vi "XYGraphView.vi"() -> ()   [LabVIEW 2014]
uses:
  GlobalData/GlobalXyData.vi
panel:
  in  "btnInitial":bool
  in  "太線(+3)":bool
  in  "自動スケール":bool
  in  "軸本数":u16(ring)=4 items=["２"=2, "４"=4, "６"=6, "８"=8]
  in  "MIN":dbl format="%#_6f"
  in  "MAX":dbl format="%#_6f"
  in  "Y軸":u16(ring) items=["No.", "M1回転rpm", "M2回転rpm", "M3回転rpm", "M1トルクN･m", "M2トルクN･m", "M3トルクN･m", "a"]
  in  "プロットCH":u16(ring) items=["No.", "M1回転rpm", "M2回転rpm", "M3回転rpm", "M1トルクN･m", "M2トルクN･m", "M3トルクN･m", "", "", "", "", "", "", "", "", "", "", "供試体温度1℃", "供試体温度2℃", "供試体温度3℃", "動力盤温度℃", "軸受温度1℃", "軸受温度2℃", "軸受温度3℃", "", "効率"]
  in  "名称":string
  in  "色":u32(colorbox)
  in  "btnAddCursor":bool
  in  "btnScaleLegendVis":bool
  in  "btnLegVis":bool
  in  "btnCursorLegendVis":bool
  out "XYグラフ":cluster{"X配列":dbl[], "Y配列":dbl[]}[](graph)
  # "表示"
  # "カーソル"
  # "グラフCH設定"
  # "右クリック→カーソルを作成→複数プロット。さらに右クリック→監視→全てのプロット"
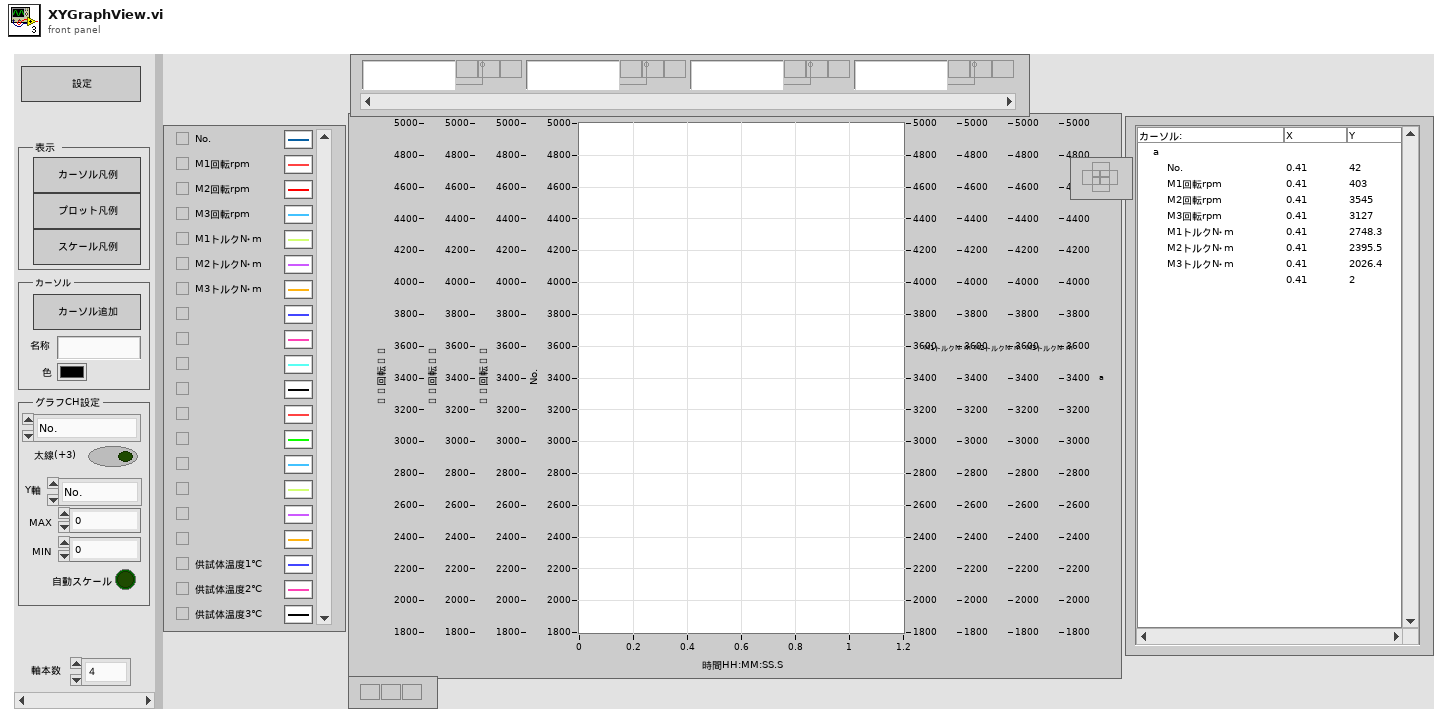
[diagram p1: front panel]
types:
  T1 = typedef "eventvkey.ctl" = enum16{"ASCII", "Enter", "Return", "Shift", "Ctrl", "Alt", "Cmd", "Opt", "Caps", "NumLock", "Clear", "Break", "Up", "Down", "Left", "Right", "Insert", "Delete", "Home", "End", "PageUp", "PageDown", "Escape", "Help", "Pause", "ScrollLock", "F1", "F2", "F3", "F4", "F5", "F6", "F7", "F8", "F9", "F10", "F11", "F12", "F13", "F14", "F15", "F16", "F17", "F18", "F19", "F20", "F21", "F22", "F23", "F24", "Play", "VolumeUp", "VolumeDown", "Mute", "Two Byte Char"}
  T2 = typedef "LVRangeTypeDef.ctl" = cluster{"Minimum":dbl, "Maximum":dbl, "Increment":dbl, "Minor Increment":dbl, "Start":dbl}
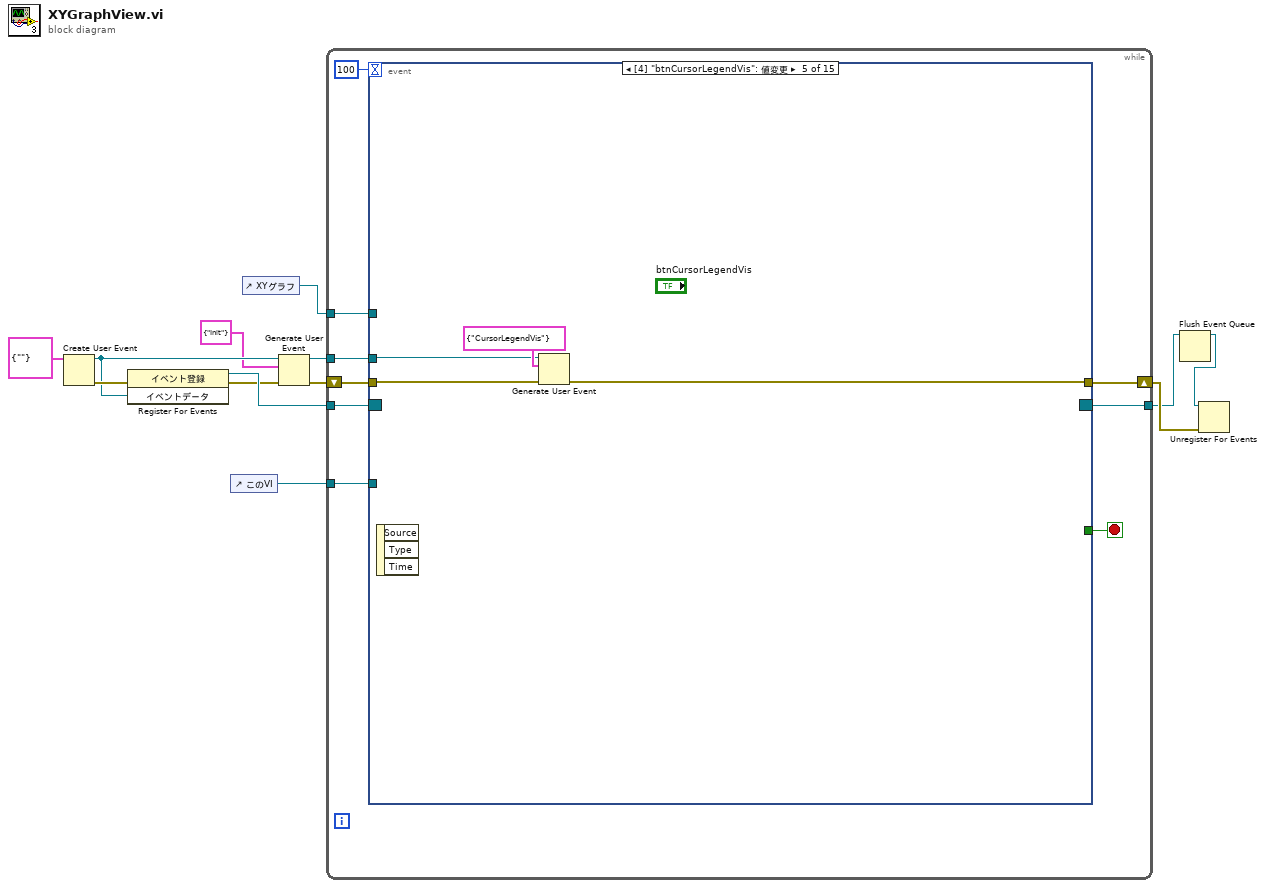
[diagram p0: block diagram]
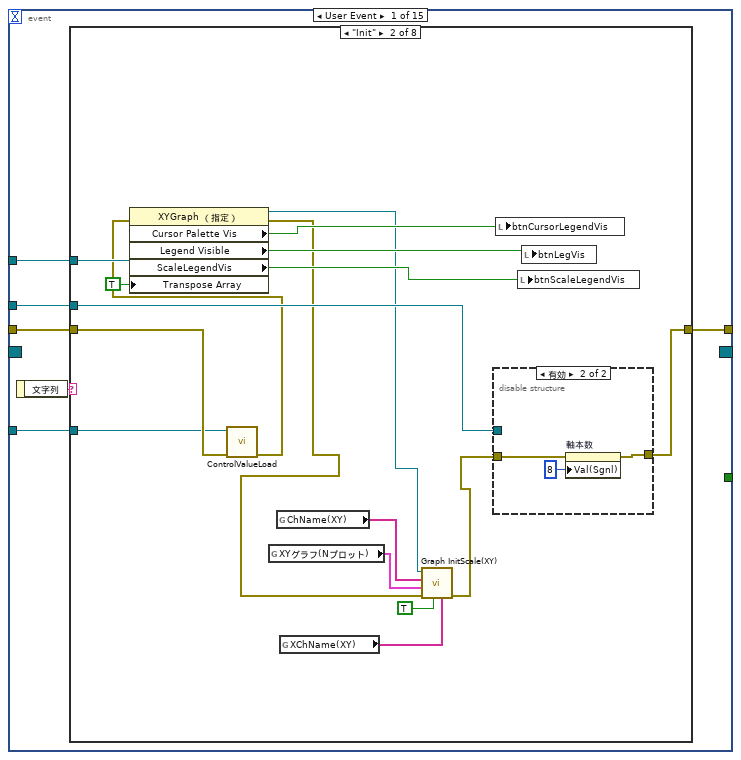
[diagram p2: hidden frame]
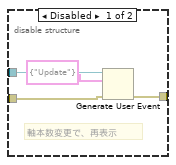
[diagram p4: hidden frame]
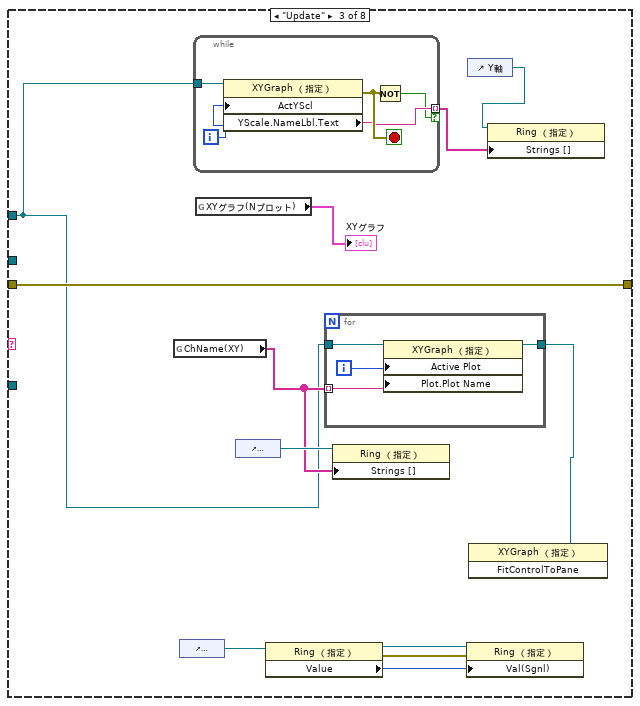
[diagram p5: hidden frame]
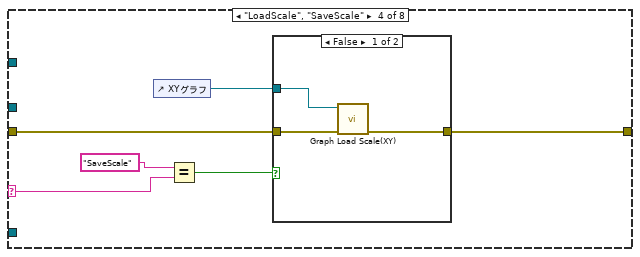
[diagram p6: hidden frame]
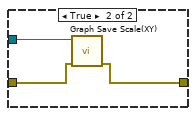
[diagram p7: hidden frame]
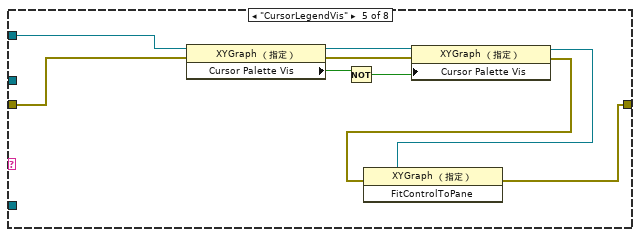
[diagram p8: hidden frame]
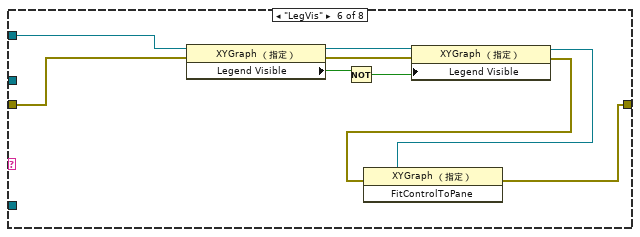
[diagram p9: hidden frame]
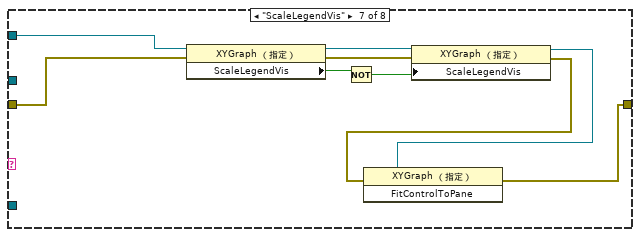
[diagram p10: hidden frame]
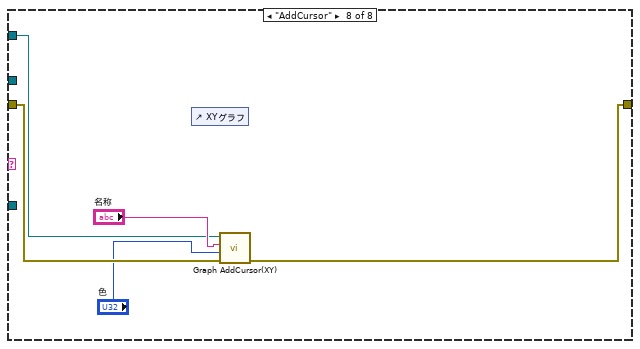
[diagram p11: hidden frame]
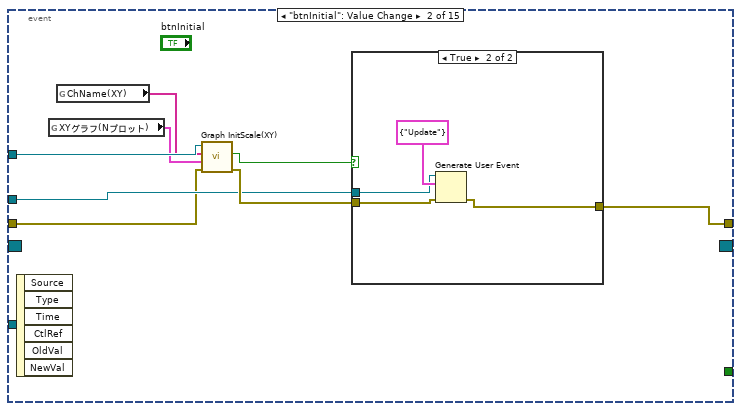
[diagram p12: hidden frame]
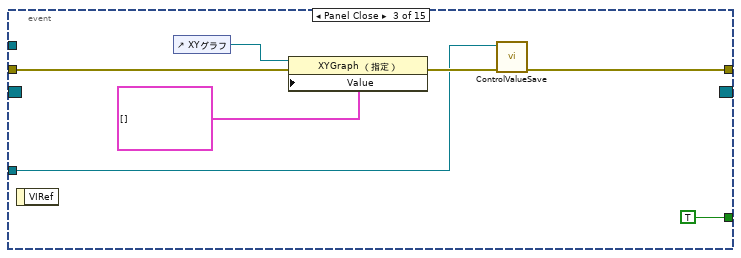
[diagram p14: hidden frame]
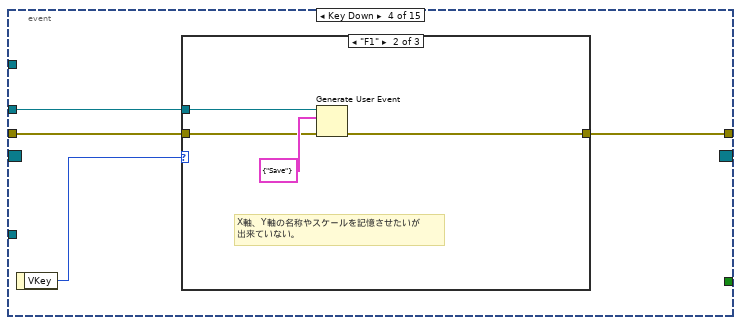
[diagram p15: hidden frame]
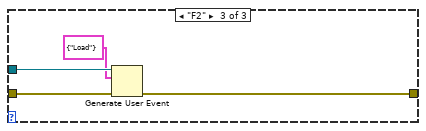
[diagram p17: hidden frame]
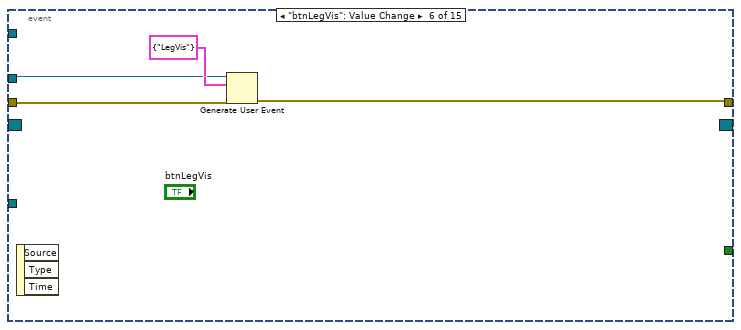
[diagram p18: hidden frame]
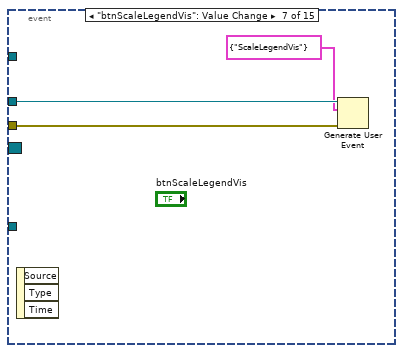
[diagram p19: hidden frame]
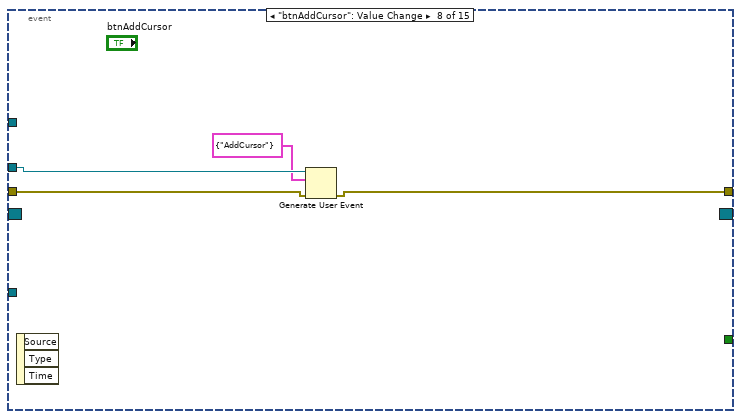
[diagram p20: hidden frame]
diagram:
  n1 = Create User Event(user event datatype=cluster{"文字列":string} {"文字列"=""} ("イベントデータ")) -> (user event=w10:refnum<user-event>, error out=w11:errorcluster)  [unwired: 1 in]
  n2 = register-events(error in=w11, w10) -> (reference out=w13:refnum<event-registration>, error out=w9:errorcluster)  [unwired: 1 in]
  n3 = control-ref of="このVI"() -> (w5:refnum<vi>)
  n4 = control-ref of="XYグラフ"() -> (w3:refnum<vi>)
  n5 = Generate User Event(user event=w10, event data cluster=cluster{"文字列":string} {"文字列"="Init"} ("イベントデータ"), error in=w9) -> (user event out=w6:refnum<user-event>, error out=w8:errorcluster)  [unwired: 1 in]
  n6 = while {
    tunnel: w13 -> [w21]
    tunnel: [w20] -> w2
    tunnel: w6 -> [w19]
    tunnel: w5 -> [w18]
    shift-right: [w16] -> w4
    shift-left: w8 -> [w17]
    tunnel: w3 -> [w15]
    stop <- w22 stop-if-true
    n7 = event shown="[4] \"btnCursorLegendVis\": 値変更" {
      selector: w21 -> [_ _ _ _ _ _ _ _ _ _ _ _ _ _ _]
      dyn-events: [_ _ _ _ _ _ _ _ _ _ _ _ _ _ _] -> w20
      timeout: 100 -> [_ _ _ _ _ _ _ _ _ _ _ _ _ _ _]
      tunnel: [_ _ TRUE _ _ _ _ _ _ _ _ _ _ _ _] -> w22
      tunnel: w19 -> [w27 w124 _ w141 w153 w158 w162 w166 _ _ _ _ w208 _ _]
      tunnel: w18 -> [w26 _ w135 _ _ _ _ _ _ _ _ _ _ _ _]
      tunnel: w17 -> [w25 w123 w137 w140 w155 w157 w160 w164 w171 _ w196 _ w207 _ w240]
      tunnel: [w24 w122 w134 w139 w152 w156 _ w163 w169 _ w189 _ w205 _ w239] -> w16
      tunnel: w15 -> [w23 w121 _ _ _ _ _ _ w173 w186 w188 w204 w211 w225 _]
      event User Event {
        n8 = event-data() -> ("文字列"=w28:string)  [unwired: 1 in]
        n9 = case shown="\"Init\"" w28 {
          selector: w28 -> [_ _ _ w76 _ _ _ _]
          tunnel: w27 -> [_ w44 _ _ _ _ _ _]
          tunnel: w26 -> [_ w43 _ _ _ _ _ _]
          tunnel: w25 -> [w29 w46 w65 w79 w91 w100 w109 w118]
          tunnel: [w29 w45 w65 w78 w88 w97 w106 w117] -> w24
          tunnel: w23 -> [_ w42 w54 _ w87 w96 w105 w114]
          frame Default {
          }
          frame "Init" {
            n10 = call "ControlValueLoad.vi"("err(in)"=w46, "VI refnum"=w43) -> ("err(out)"=w38:errorcluster)  [unwired: 9 in]
            n11 = property class="XYGraph （指定）"(reference=w42, error in=w38, "Transpose Array"=TRUE ("配列転置")) -> (reference out=w30:refnum<vi>, error out=w34:errorcluster, "Cursor Palette Vis"=w41:bool, "Legend Visible"=w40:bool, "ScaleLegendVis"=w39:bool)
            n12 = global read "GlobalXyData.vi" "XYグラフ(Nプロット)"() -> (w35:cluster{"X配列":dbl[], "Y配列":dbl[]}[])
            n13 = global read "GlobalXyData.vi" "ChName(XY)"() -> (w36:string[])
            n14 = global read "GlobalXyData.vi" "XChName(XY)"() -> (w31:string[])
            n15 = call "Graph InitScale(XY).vi"("XChName(XY)"=w31, "初回?"=TRUE, "error in (no error)"=w34, "XYグラフ(Nプロット)"=w35, "ChName(XY)"=w36, "XYグラフ(ref)"=w30) -> ("error out"=w33:errorcluster)  [unwired: 4 in, 1 out]
            n16 = disable-structure shown="有効" {
              disable-tunnel: [w50 w52] -> w45
              disable-tunnel: w44 -> [w49 _]
              disable-tunnel: w33 -> [w47 w53]
              frame Disabled {
                # "軸本数変更で、再表示"
                n17 = Generate User Event(user event=w49, event data cluster=cluster{"文字列":string} {"文字列"="Update"} ("イベントデータ"), error in=w47) -> (error out=w50:errorcluster)  [unwired: 1 in, 1 out]
              }
              frame Enabled {
                n18 = property on="軸本数" class="Ring （指定）"(error in=w53, "Val(Sgnl)"=u16 8 ("値（信号）")) -> (error out=w52:errorcluster)  [unwired: 1 in, 1 out]
              }
            }
            n19 = local write "btnCursorLegendVis"(w41) -> ()
            n20 = local write "btnScaleLegendVis"(w39) -> ()
            n21 = local write "btnLegVis"(w40) -> ()
          }
          frame "Update" {
            n22 = global read "GlobalXyData.vi" "ChName(XY)"() -> (w59:string[])
            n23 = control-ref of="プロットCH"() -> (w58:refnum<vi>)
            n24 = while {
              tunnel: w54 -> [w70]
              tunnel: [w67] -> w62 mode=indexing if=w66
              i -> [w69]
              stop <- w68 stop-if-true
              n25 = property class="XYGraph （指定）"(reference=w70, "ActYScl"=w69) -> (error out=w68:errorcluster, "YScale.NameLbl.Text"=w67:string)  [unwired: 1 in, 1 out]
              n26 = Not(x=w68) -> (.not. x?=w66:bool)
            }
            n27 = global read "GlobalXyData.vi" "XYグラフ(Nプロット)"() -> (→"XYグラフ":cluster{"X配列":dbl[], "Y配列":dbl[]}[])
            n28 = control-ref of="プロットCH"() -> (w64:refnum<vi>)
            n29 = property class="Ring （指定）"(reference=w58) -> (reference out=w56:refnum<vi>, error out=w55:errorcluster, "Value"=w57:u16)  [unwired: 1 in]
            n30 = for {
              tunnel: w54 -> [w74]
              tunnel: w59 -> [w73] mode=indexing
              tunnel: [w71] -> w61
              i -> [w72]
              n31 = property class="XYGraph （指定）"(reference=w74, "Active Plot"=w72, "Plot.Plot Name"=w73) -> (reference out=w71:refnum<vi>)  [unwired: 1 in, 1 out]
            }
            n32 = property class="Ring （指定）"(reference=w64, "Strings []"=w59) -> ()  [unwired: 1 in, 2 out]
            n33 = property class="Ring （指定）"(reference=w56, error in=w55, "Val(Sgnl)"=w57) -> ()  [unwired: 2 out]
            n34 = control-ref of="Y軸"() -> (w63:refnum<vi>)
            n35 = invoke class="XYGraph （指定）" method="FitControlToPane"(reference=w61) -> ()  [unwired: 2 in, 3 out]
            n36 = property class="Ring （指定）"(reference=w63, "Strings []"=w62) -> ()  [unwired: 1 in, 2 out]
          }
          frame "LoadScale", "SaveScale" {
            n37 = control-ref of="XYグラフ"() -> (w80:refnum<vi>)
            n38 = Equal?(x="SaveScale", y=w76) -> (x = y?=w75:bool)
            n39 = case shown="FALSE" w75 {
              tunnel: w80 -> [w83 w86]
              tunnel: w79 -> [w82 w85]
              tunnel: [w81 w84] -> w78
              frame False {
                n40 = call "Graph Load Scale(XY).vi"("err in"=w82, "XYGraph入力"=w83) -> ("err out"=w81:errorcluster)  [unwired: 9 in]
              }
              frame True {
                n41 = call "Graph Save Scale(XY).vi"("err in"=w85, "WaveformGraph入力"=w86) -> ("error out"=w84:errorcluster)  [unwired: 9 in]
              }
            }
          }
          frame "CursorLegendVis" {
            n42 = property class="XYGraph （指定）"(reference=w87, error in=w91) -> (reference out=w92:refnum<vi>, error out=w93:errorcluster, "Cursor Palette Vis"=w95:bool)
            n43 = Not(x=w95) -> (.not. x?=w94:bool)
            n44 = property class="XYGraph （指定）"(reference=w92, error in=w93, "Cursor Palette Vis"=w94) -> (reference out=w90:refnum<vi>, error out=w89:errorcluster)
            n45 = invoke class="XYGraph （指定）" method="FitControlToPane"(reference=w90, error in=w89) -> (error out=w88:errorcluster)  [unwired: 1 in, 2 out]
          }
          frame "LegVis" {
            n46 = property class="XYGraph （指定）"(reference=w96, error in=w100) -> (reference out=w101:refnum<vi>, error out=w102:errorcluster, "Legend Visible"=w104:bool)
            n47 = Not(x=w104) -> (.not. x?=w103:bool)
            n48 = property class="XYGraph （指定）"(reference=w101, error in=w102, "Legend Visible"=w103) -> (reference out=w99:refnum<vi>, error out=w98:errorcluster)
            n49 = invoke class="XYGraph （指定）" method="FitControlToPane"(reference=w99, error in=w98) -> (error out=w97:errorcluster)  [unwired: 1 in, 2 out]
          }
          frame "ScaleLegendVis" {
            n50 = property class="XYGraph （指定）"(reference=w105, error in=w109) -> (reference out=w110:refnum<vi>, error out=w111:errorcluster, "ScaleLegendVis"=w113:bool)
            n51 = Not(x=w113) -> (.not. x?=w112:bool)
            n52 = property class="XYGraph （指定）"(reference=w110, error in=w111, "ScaleLegendVis"=w112) -> (reference out=w108:refnum<vi>, error out=w107:errorcluster)
            n53 = invoke class="XYGraph （指定）" method="FitControlToPane"(reference=w108, error in=w107) -> (error out=w106:errorcluster)  [unwired: 1 in, 2 out]
          }
          frame "AddCursor" {
            n54 = control-ref of="XYグラフ"() -> ()  [unwired: 1 out]
            n55 = call "Graph AddCursor(XY).vi"("エラー入力（エラーなし）"=w118, "色"="色", "名称"="名称", "XYグラフref"=w114) -> ("エラー出力"=w117:errorcluster)  [unwired: 7 in]
          }
        }
      }
      event "btnInitial": Value Change {
        n56 = event-data() -> ()  [unwired: 1 in, 6 out]
        n57 = global read "GlobalXyData.vi" "XYグラフ(Nプロット)"() -> (w119:cluster{"X配列":dbl[], "Y配列":dbl[]}[])
        n58 = global read "GlobalXyData.vi" "ChName(XY)"() -> (w120:string[])
        n59 = call "Graph InitScale(XY).vi"("error in (no error)"=w123, "XYグラフ(Nプロット)"=w119, "ChName(XY)"=w120, "XYグラフ(ref)"=w121) -> ("error out"=w125:errorcluster, "OK"=w126:bool)  [unwired: 6 in]
        n60 = case shown="TRUE" w126 {
          tunnel: w124 -> [_ w130]
          tunnel: w125 -> [w127 w129]
          tunnel: [w127 w128] -> w122
          frame False {
          }
          frame True {
            n61 = Generate User Event(user event=w130, event data cluster=cluster{"文字列":string} {"文字列"="Update"} ("イベントデータ"), error in=w129) -> (error out=w128:errorcluster)  [unwired: 1 in, 1 out]
          }
        }
      }
      event Panel Close {
        n62 = event-data() -> ()  [unwired: 1 in, 1 out]
        n63 = control-ref of="XYグラフ"() -> (w133:refnum<vi>)
        n64 = property class="XYGraph （指定）"(reference=w133, error in=w137, "Value"=cluster{"X配列":dbl[], "Y配列":dbl[]}[] [] ("値")) -> (error out=w136:errorcluster)  [unwired: 1 out]
        n65 = call "ControlValueSave.vi"("err(in)"=w136, "VI refnum"=w135) -> ("err(out)"=w134:errorcluster)  [unwired: 9 in]
      }
      event Key Down {
        n66 = event-data() -> ("VKey"=w142:T1)  [unwired: 1 in]
        n67 = case shown="\"F1\"" w142 {
          tunnel: w141 -> [_ w147 w151]
          tunnel: w140 -> [w143 w145 w149]
          tunnel: [w143 w144 w148] -> w139
          frame "ASCII", Default {
          }
          frame "F1" {
            # "X軸、Y軸の名称やスケールを記憶させたいが\n出来ていない。"
            n68 = Generate User Event(user event=w147, event data cluster=cluster{"文字列":string} {"文字列"="Save"} ("イベントデータ"), error in=w145) -> (error out=w144:errorcluster)  [unwired: 1 in, 1 out]
          }
          frame "F2" {
            n69 = Generate User Event(user event=w151, event data cluster=cluster{"文字列":string} {"文字列"="Load"} ("イベントデータ"), error in=w149) -> (error out=w148:errorcluster)  [unwired: 1 in, 1 out]
          }
        }
      }
      event "btnCursorLegendVis": Value Change {
        n70 = event-data() -> ()  [unwired: 1 in, 3 out]
        n71 = Generate User Event(user event=w153, event data cluster=cluster{"文字列":string} {"文字列"="CursorLegendVis"} ("イベントデータ"), error in=w155) -> (error out=w152:errorcluster)  [unwired: 1 in, 1 out]
      }
      event "btnLegVis": Value Change {
        n72 = event-data() -> ()  [unwired: 1 in, 3 out]
        n73 = Generate User Event(user event=w158, event data cluster=cluster{"文字列":string} {"文字列"="LegVis"} ("イベントデータ"), error in=w157) -> (error out=w156:errorcluster)  [unwired: 1 in, 1 out]
      }
      event "btnScaleLegendVis": Value Change {
        n74 = event-data() -> ()  [unwired: 1 in, 3 out]
        n75 = Generate User Event(user event=w162, event data cluster=cluster{"文字列":string} {"文字列"="ScaleLegendVis"} ("イベントデータ"), error in=w160) -> ()  [unwired: 1 in, 2 out]
      }
      event "btnAddCursor": Value Change {
        n76 = event-data() -> ()  [unwired: 1 in, 3 out]
        n77 = Generate User Event(user event=w166, event data cluster=cluster{"文字列":string} {"文字列"="AddCursor"} ("イベントデータ"), error in=w164) -> (error out=w163:errorcluster)  [unwired: 1 in, 1 out]
      }
      event "プロットCH": Value Change {
        n78 = event-data() -> ()  [unwired: 1 in, 1 out]
        n79 = property class="XYGraph （指定）"(reference=w173, error in=w171, "Active Plot"="プロットCH") -> (reference out=w170:refnum<vi>, error out=w169:errorcluster, "Plot.YScaleIdx"=w168:u32)
        n80 = To Unsigned Word Integer(number=w168) -> (unsigned 16bit integer=w176:u16)
        n81 = property class="XYGraph （指定）"(reference=w170, error in=w169, "ActYScl"=w168) -> ("YScale.Range"=w167:T2)  [unwired: 2 out]
        n82 = local write "Y軸"(w176) -> ()
        n83 = Unbundle By Name(w167) -> ("Maximum"=w175:dbl, "Minimum"=w174:dbl)
        n84 = local write "MIN"(w174) -> ()
        n85 = local write "MAX"(w175) -> ()
      }
      event "Y軸": Value Change {
        n86 = event-data() -> ()  [unwired: 1 in, 6 out]
        n87 = local read "プロットCH"() -> (w185:u16)
        n88 = property class="XYGraph （指定）"(reference=w186, "Active Plot"=w185) -> (reference out=w179:refnum<vi>, error out=w183:errorcluster, "Plot"=w184:refnum<vi>)  [unwired: 1 in]
        n89 = property class="Plot"(reference=w184, error in=w183, "YScaleIdx"="Y軸") -> (error out=w177:errorcluster)  [unwired: 1 out]
        n90 = property class="XYGraph （指定）"(reference=w179, error in=w177, "ActYScl"="Y軸") -> ("YScale.Range"=w182:T2)  [unwired: 2 out]
        n91 = Unbundle By Name(w182) -> ("Maximum"=w181:dbl, "Minimum"=w180:dbl)
        n92 = local write "MAX"(w181) -> ()
        n93 = local write "MIN"(w180) -> ()
      }
      event "MAX", "MIN": Value Change {
        n94 = event-data() -> ()  [unwired: 1 in, 6 out]
        n95 = local read "Y軸"() -> (w187:u16)
        n96 = property class="XYGraph （指定）"(reference=w188, error in=w196, "ActYScl"=w187) -> (reference out=w194:refnum<vi>, error out=w192:errorcluster, "YScale.Range"=w195:T2)
        n97 = Bundle By Name(cluster=w195, "Maximum"="MAX", "Minimum"="MIN") -> (w193:T2)
        n98 = property class="XYGraph （指定）"(reference=w194, error in=w192, "YScale.Range"=w193) -> (error out=w189:errorcluster)  [unwired: 1 out]
      }
      event "自動スケール": Value Change {
        n99 = event-data() -> ()  [unwired: 1 in, 6 out]
        n100 = local read "Y軸"() -> (w203:u16)
        n101 = property class="XYGraph （指定）"(reference=w204, "ActYScl"=w203, "YScale.ScaleFit"=u8 1 ("Yスケール.スケールフィット")) -> (reference out=w201:refnum<vi>, error out=w200:errorcluster)  [unwired: 1 in]
        n102 = property class="XYGraph （指定）"(reference=w201, error in=w200) -> ("YScale.Range"=w199:T2)  [unwired: 2 out]
        n103 = Unbundle By Name(w199) -> ("Maximum"=w198:dbl, "Minimum"=w197:dbl)
        n104 = local write "MAX"(w198) -> ()
        n105 = local write "MIN"(w197) -> ()
      }
      event "軸本数": Value Change {
        n106 = event-data() -> ()  [unwired: 1 in, 6 out]
        n107 = while {
          tunnel: w211 -> [w219]
          tunnel: [w213] -> w210
          tunnel: w207 -> [w212]
          i -> [w218]
          stop <- w214 stop-if-true
          n108 = To Unsigned Word Integer(number=w218) -> (unsigned 16bit integer=w215:u16)
          n109 = Less?(x=w215, y="軸本数") -> (x < y?=w216:bool)
          n110 = property class="XYGraph （指定）"(reference=w219, error in=w212, "ActYScl"=w218, "YScale.Visible"=w216) -> (reference out=w213:refnum<vi>, error out=w214:errorcluster)
        }
        n111 = invoke class="XYGraph （指定）" method="FitControlToPane"(reference=w210) -> (error out=w206:errorcluster)  [unwired: 2 in, 2 out]
        n112 = Generate User Event(user event=w208, event data cluster=cluster{"文字列":string} {"文字列"="Update"} ("イベントデータ"), error in=w206) -> (error out=w205:errorcluster)  [unwired: 1 in, 1 out]
      }
      event Timeout {
        n113 = event-data() -> ()  [unwired: 1 in, 3 out]
        n114 = local read "プロットCH"() -> (w224:u16)
        n115 = feedback-in #1("太線(+3)") -> ()
        n116 = feedback #1() -> (w228:bool)  [unwired: 1 in]
        n117 = Build Array("太線(+3)", w228) -> (w227:bool[])
        n118 = property class="XYGraph （指定）"(reference=w225, "Active Plot"=w224) -> (reference out=w222:refnum<vi>, "Plot.Line Width"=w223:u8)  [unwired: 1 in, 1 out]
        n119 = Boolean Array To Number(Boolean array=w227) -> (number=w226:u32)
        n120 = case shown="1" w226 {
          tunnel: w223 -> [_ w231 w236]
          tunnel: w222 -> [_ w233 w238]
          tunnel: 3 -> [_ w230 w235]
          frame 0, Default {
          }
          frame 2 {
            # "ON->OFF"
            n121 = Subtract(x=w231, y=w230) -> (x-y=w229:i32)
            n122 = To Unsigned Byte Integer(number=w229) -> (unsigned 8bit integer=w232:u8)
            n123 = property class="XYGraph （指定）"(reference=w233, "Plot.Line Width"=w232) -> ()  [unwired: 1 in, 2 out]
          }
          frame 1 {
            # "OFF->ON"
            n124 = Add(x=w236, y=w235) -> (x+y=w234:i32)
            n125 = To Unsigned Byte Integer(number=w234) -> (unsigned 8bit integer=w237:u8)
            n126 = property class="XYGraph （指定）"(reference=w238, "Plot.Line Width"=w237) -> ()  [unwired: 1 in, 2 out]
          }
        }
      }
      event "XYグラフ": Plot Attribute Change {
        n127 = event-data() -> ("PlotIdx"=w241:i32)  [unwired: 1 in, 7 out]
        n128 = property on="プロットCH" class="Ring （指定）"(error in=w240, "Val(Sgnl)"=w241) -> (error out=w239:errorcluster)  [unwired: 1 in, 1 out]
      }
    }
  }
  n129 = Flush Event Queue(0:w2) -> (8:w1:refnum<event-registration>)  [unwired: 5 in, 2 out]
  n130 = Unregister For Events(event registration refnum=w1, error in=w4) -> ()  [unwired: 1 out]
